vi "Untitled 2.vi"() -> ()   [LabVIEW 2017]
uses:
  <vilib>/myRIO/Common/Instrument Driver Framework/myRIO v1.0/Encoder/typedefs/Encoder Signal Mode.ctl
  <vilib>/myRIO/Instrument Drivers/Onboard IO/Encoder/typedefs/Encoder Reference.ctl
  <vilib>/myRIO/Common/Instrument Driver Framework/Utilities/typedefs/myRIO Generic Hardware Reference.ctl
  <vilib>/myRIO/Common/Instrument Driver Framework/Utilities/typedefs/Hardware Version Enum.ctl
  <vilib>/myRIO/Common/Instrument Driver Framework/Utilities/typedefs/myRIO v1.0 Reference.ctl
  <vilib>/myRIO/Common/Instrument Driver Framework/Utilities/typedefs/Generic FPGA Reference.ctl
  <vilib>/myRIO/Common/Instrument Driver Framework/myRIO v1.0/Encoder/typedefs/Encoder Channels Enum.ctl
  <vilib>/myRIO/Common/Instrument Driver Framework/myRIO v1.0/Encoder/typedefs/Encoder Configuration v1.0.ctl
  <vilib>/userdefined/High Color/nirio_resource_hc.ctl
  <vilib>/myRIO/Common/Instrument Driver Framework/Utilities/vis/Is FPGA Ref Available.vi
  <vilib>/myRIO/Common/Instrument Driver Framework/myRIO v1.0/Encoder/vis/myRIO v1.1 Open Encoder.vi
  <vilib>/myRIO/Instrument Drivers/Onboard IO/Encoder/vis/Read.vi
  <vilib>/myRIO/Common/Instrument Driver Framework/Utilities/vis/Validate Channels.vi
  <vilib>/myRIO/Common/Instrument Driver Framework/myRIO v1.0/Encoder/vis/myRIO v1.0 Reserve Encoder.vi
  <vilib>/myRIO/Common/Instrument Driver Framework/myRIO v1.0/Encoder/vis/myRIO v1.0 Build MUX Configuration Encoder.vi
  <vilib>/myRIO/Common/Instrument Driver Framework/myRIO v1.0/Resource Manager/vis/myRIO v1.0 Reserve Channel List.vi
  <vilib>/myRIO/Common/Instrument Driver Framework/myRIO v1.0/Resource Manager/vis/myRIO v1.0 Create Configuration List.vi
  <vilib>/myRIO/Common/Instrument Driver Framework/myRIO v1.0/Resource Manager/vis/myRIO v1.0 Reserve Channel.vi
  <vilib>/myRIO/Common/Instrument Driver Framework/myRIO v1.0/Resource Manager/vis/myRIO v1.0 Unreserve Channel.vi
  <vilib>/myRIO/Common/Instrument Driver Framework/myRIO v1.0/Resource Manager/vis/myRIO v1.0 Build Mutex Name.vi
  <vilib>/Utility/VariantDataType/GetNumericInfo.vi
  <vilib>/Utility/error.llb/Error Cluster From Error Code.vi
  <vilib>/myRIO/Common/Instrument Driver Framework/myRIO v1.0/myRIO v1.1 Open.vi
  <vilib>/myRIO/Common/Instrument Driver Framework/Utilities/vis/IO Manager.vi
  <vilib>/myRIO/Common/Instrument Driver Framework/Utilities/vis/Configuration Manager.vi
  <vilib>/myRIO/Common/Instrument Driver Framework/myRIO v1.0/Resource Manager/vis/myRIO v1.0 Configure IO.vi
  <vilib>/myRIO/Common/Instrument Driver Framework/myRIO v1.0/myRIO v1.0 Close.vi
  <vilib>/myRIO/Common/Instrument Driver Framework/myRIO v1.0/Encoder/vis/myRIO v1.0 Configure Encoder.vi
  <vilib>/myRIO/Common/Instrument Driver Framework/myRIO v1.0/Encoder/vis/myRIO v1.0 Read Encoder.vi
  <vilib>/addons/control/pid/pid.llb/PID (DBL).vi
  <vilib>/myRIO/Express VI/Onboard IO/Encoder/Encoder Express VI.xnode
  <vilib>/myRIO/Instrument Drivers/Onboard IO/Encoder/vis/myRIO Encoder Open.xnode
  <vilib>/myRIO/Common/Instrument Driver Framework/myRIO v1.0/Encoder/typedefs/Encoder Count Direction Enum.ctl
  <vilib>/addons/control/pid/NI_PID_pid.lvlib
  <vilib>/myRIO/Instrument Drivers/Onboard IO/Encoder/Encoder.lvlib
panel:
  in  "Min Speed":dbl=1.0
  in  "Max Speed":dbl=3.0
  out "PID B":T1(graph)={"Setpoint"=1.9492814755476044, "output"=0.04903176938944572, "dx/dt"=3.0}
  out "PID A":T1(graph)={"Setpoint"=1.7890362814617413, "output"=0.16204700765601243, "dx/dt"=0.9259999999994761}
  out "OUTPUT A":dbl(slide)=0.9259999999994761 scale=-10.0..10.0
  out "OUTPUT B":dbl(slide)=3.0 scale=-10.0..10.0
  in  "stop":bool=TRUE
  in  "PID gains":T2={"proportional gain (Kc)"=0.04, "integral time (Ti, min)"=0.1, "derivative time (Td, min)"=0.0} {"derivative time (Td, min)" format="%.3f"; "integral time (Ti, min)" format="%.3f"; "proportional gain (Kc)" format="%.3f"}
  out "XY Graph":cluster{"X":dbl, "Y":dbl}[](graph)=[{"X"=-30.082698286482174, "Y"=7953.93623198267}, {"X"=-30.068060606349714, "Y"=7954.135185370846}]
  in  "speed":dbl(slide)=1.8691588785046729 scale=0.0..10.0
  in  "angle":dbl(slide) scale=-90.0..90.0
  out "Waveform Chart":dbl(graph)=4.207864617948657
  in  "Initial X, Y, BEARING":cluster{dbl, dbl, dbl}
  out "Final X, Y, BEARING":cluster{dbl, dbl, dbl}={-30.068060606349714, 7954.135185370846, 4.207864617948657}
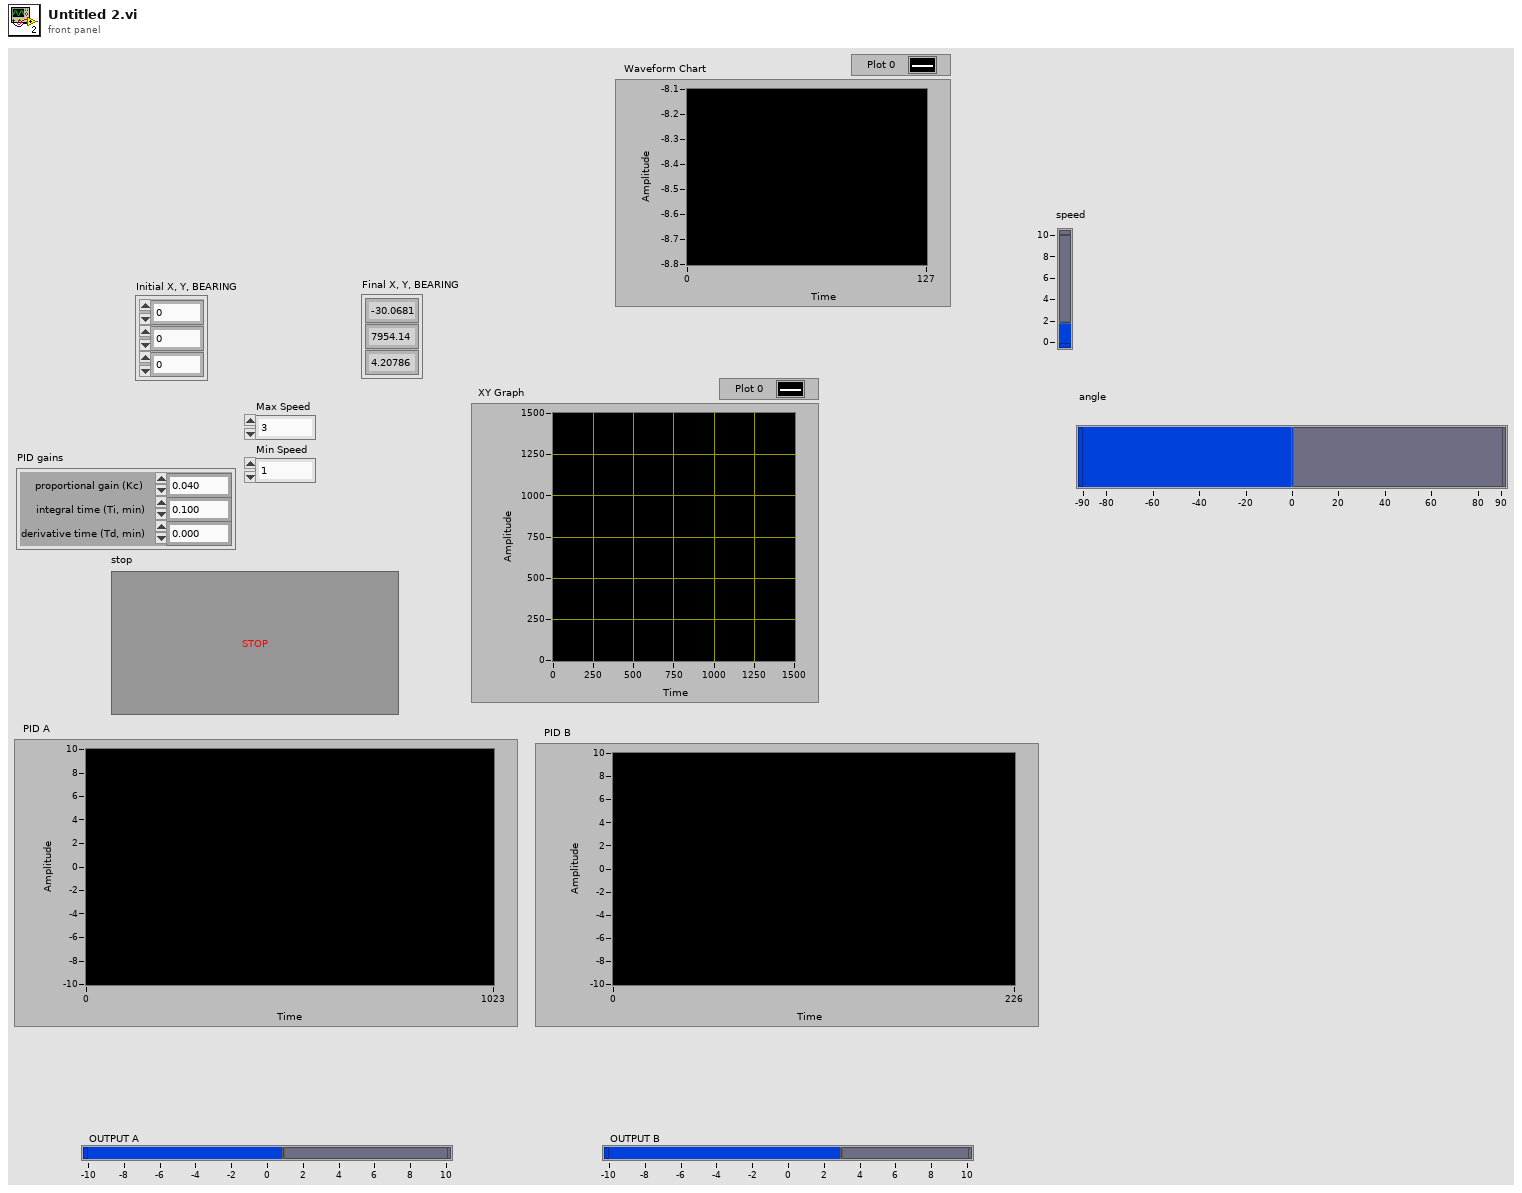
[diagram p1: front panel]
types:
  T1 = cluster{"Setpoint":dbl, "output":dbl, "dx/dt":dbl}
  T2 = cluster{"proportional gain (Kc)":dbl, "integral time (Ti, min)":dbl, "derivative time (Td, min)":dbl}
  T3 = cluster{"Strength":dbl, "Distance from Wall":dbl}
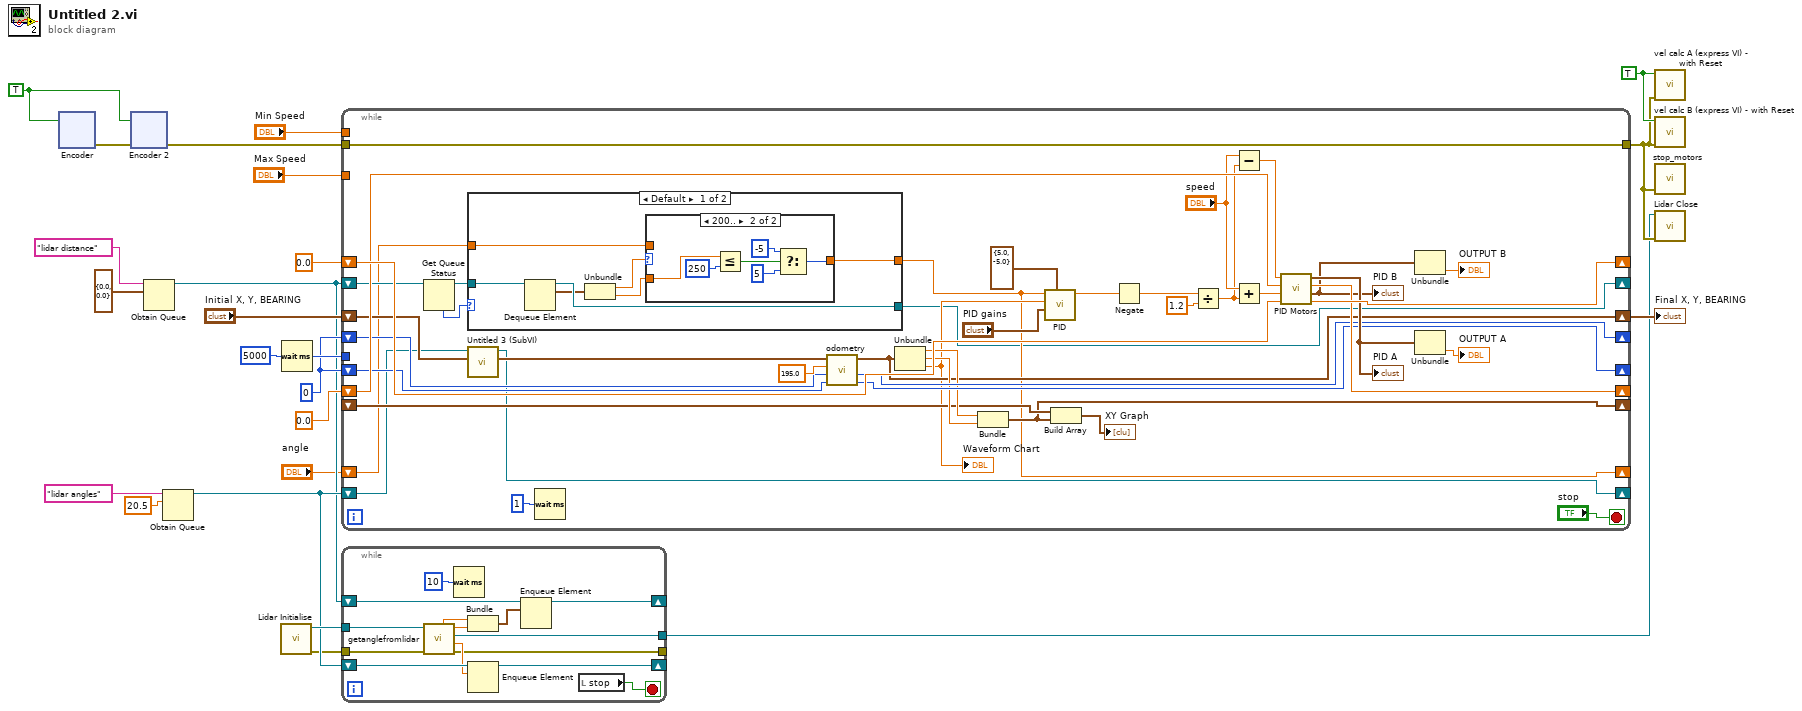
[diagram p0: block diagram]
diagram:
  w12 = TRUE ("Reinitialise")
  w14 = TRUE
  w18 = 0 ("ENCA OUT")
  n1 = xnode "Encoder"("Reset Counter"=w14) -> ("error out"=w15:errorcluster)  [unwired: 1 in, 3 out]
  n2 = xnode "Encoder 2"("error in (no error)"=w15, "Reset Counter"=w14) -> ("error out"=w13:errorcluster)  [unwired: 3 out]
  n3 = Obtain Queue(name (unnamed)="lidar distance", element data type=T3 {"Strength"=0.0, "Distance from Wall"=0.0} ("output cluster")) -> (queue out=w2:refnum<queue>)  [unwired: 3 in, 2 out]
  n4 = Obtain Queue(name (unnamed)="lidar angles", element data type=20.5) -> (queue out=w9:refnum<queue>)  [unwired: 3 in, 2 out]
  n5 = call "Lidar Initialise.vi"() -> ("error out"=w6:errorcluster, "VISA resource name out"=w11:refnum<visa-resource-name>)  [unwired: 10 in]
  n6 = Wait (ms)(milliseconds to wait=u32 5000) -> (millisecond timer value=w22:u32)
  n7 = while {
    tunnel: w13 -> [w60]
    shift-right: [w62] -> _
    shift-left: 0.0 ("output A") -> [w63]
    shift-right: [w65] -> _
    shift-left: 0.0 ("output B") -> [w64]
    tunnel: [w60] -> w8
    shift-right: [w52] -> _
    shift-left: w18 -> [w54]
    shift-right: [w51] -> _
    shift-left: w18 -> [w53]
    shift-right: [w39] -> w24
    shift-left: "Initial X, Y, BEARING" -> [w43]
    shift-right: [w47] -> _
    shift-left: _ -> [w48]
    tunnel: "Max Speed" -> [_]
    tunnel: "Min Speed" -> [_]
    tunnel: w22 -> [_]
    shift-right: [w40] -> _
    shift-left: w9 -> [w41]
    shift-right: [w27] -> _
    shift-left: "angle" -> [w28]
    shift-right: [w25] -> _
    shift-left: w2 -> [w30]
    stop <- "stop" stop-if-true
    n8 = Get Queue Status(queue=w30) -> (queue out=w26:refnum<queue>, # elements in queue=w29:i32)  [unwired: 2 in, 6 out]
    n9 = case shown="Default" w29 {
      tunnel: w28 -> [w68 w82]
      tunnel: [w67 w82] -> w27
      tunnel: w26 -> [w73 w81]
      tunnel: [w72 w81] -> w25
      frame Default {
        n10 = Dequeue Element(queue=w73) -> (queue out=w72:refnum<queue>, element=w71:T3)  [unwired: 2 in, 2 out]
        n11 = Unbundle(w71) -> ("Strength"=w70:dbl, "Distance from Wall"=w69:dbl)
        n12 = case shown="200.." w70 {
          tunnel: w69 -> [_ w79]
          tunnel: w68 -> [w74 _]
          tunnel: [w74 w75] -> w67
          frame 0, Default {
          }
          frame 200.. {
            n13 = Less Or Equal?(x=w79, y=250) -> (x <= y?=w80:bool)
            n14 = Select(t=-5, s=w80, f=5) -> (s? t:f=w75:i32)
          }
        }
      }
      frame 0 {
      }
    }
    n15 = call "Untitled 3 (SubVI).vi"("X, Y, BEARING in"=w43, "Queue in"=w41) -> ("X, Y, BEARING out"=w42:cluster{dbl, dbl, dbl}, "Queue out"=w40:refnum<queue>)  [unwired: 8 in]
    n16 = Wait (ms)(milliseconds to wait=1 ("ENCB OUT")) -> ()  [unwired: 1 out]
    n17 = call "odometry.vi"("ENCB in"=w53, "ENCA in"=w54, "wheelbase"=195.0, "Position"=w42) -> ("ENCB OUT"=w51:i32, "ENCA OUT"=w52:i32, "X, Y, BEARING"=w39:cluster{dbl, dbl, dbl})  [unwired: 4 in]
    n18 = Unbundle(w39) -> (w49:dbl, w50:dbl, w35:dbl)
    "Waveform Chart" <- w35
    n19 = Bundle(w49, w50) -> (w47:cluster{dbl, dbl})  [unwired: 1 in]
    n20 = call-poly <vilib>:"PID.vi"("output range"=cluster{"output high":dbl, "output low":dbl} {"output high"=5.0, "output low"=-5.0}, "PID gains"="PID gains", "process variable"=w35, "setpoint"=w27) -> ("output"=w32:dbl)  [unwired: 6 in, 1 out]
    n21 = Build Array(w48, w47) -> (→"XY Graph":cluster{dbl, dbl}[])
    n22 = Negate(x=w32) -> (-x=w31:dbl)
    n23 = Divide(x=w31, y=1.2) -> (x/y=w34:dbl)
    n24 = Subtract(x="speed", y=w34) -> (x-y=w37:dbl)
    n25 = Add(x="speed", y=w34) -> (x+y=w36:dbl)
    n26 = call "PID Motors.vi"("input B"=w64, "Speed B"=w36, "input A"=w63, "Speed A"=w37) -> ("output B"=w65:dbl, "Speed B0"=w58:T1, "output A"=w62:dbl, "Speed A0"=w59:T1)
    "PID B" <- w58
    "PID A" <- w59
    n27 = Unbundle(w58) -> ("dx/dt"=→"OUTPUT B":dbl)  [unwired: 2 out]
    n28 = Unbundle(w59) -> ("dx/dt"=→"OUTPUT A":dbl)  [unwired: 2 out]
  }
  "Final X, Y, BEARING" <- w24
  n29 = while {
    tunnel: w11 -> [w96]
    shift-right: [w92] -> _
    shift-left: w9 -> [w94]
    tunnel: [w91] -> w7
    tunnel: w6 -> [w90]
    tunnel: [w89] -> _
    shift-right: [w84] -> _
    shift-left: w2 -> [w85]
    stop <- w95 stop-if-true
    n30 = call "getanglefromlidar.vi"("error in (no error)"=w90, "VISA resource name"=w96) -> ("error constant"=w89:errorcluster, "Angle From WALL"=w93:dbl, "VISA resource name out"=w91:refnum<visa-resource-name>, "Distance from Wall"=w86:dbl, "Strength"=w87:dbl)  [unwired: 4 in, 1 out]
    n31 = Wait (ms)(milliseconds to wait=10 ("ENCB OUT")) -> ()  [unwired: 1 out]
    n32 = Bundle("Strength"=w87, "Distance from Wall"=w86) -> (w83:T3)  [unwired: 1 in]
    n33 = Enqueue Element(queue=w94, element=w93) -> (queue out=w92:refnum<queue>)  [unwired: 2 in, 2 out]
    n34 = Enqueue Element(queue=w85, element=w83) -> (queue out=w84:refnum<queue>)  [unwired: 2 in, 2 out]
    n35 = local read "stop"() -> (w95:bool)
  }
  n36 = call "vel calc A (express VI) - with Reset.vi"("error in"=w8, "Reinitialise"=w12) -> ()  [unwired: 5 in, 5 out]
  n37 = call "vel calc B (express VI) - with Reset.vi"("error in"=w8, "Reinitialise"=w12) -> ()  [unwired: 5 in, 5 out]
  n38 = call "stop_motors.vi"("error in (no error)"=w8) -> ()  [unwired: 4 in, 1 out]
  n39 = call "Lidar Close.vi"("error in (no error)"=w8, "VISA resource name"=w7) -> ()  [unwired: 9 in, 1 out]
